vi "Open Base System Definition.vi"(8 "error in (no error)":errorcluster) -> (0 "error out":errorcluster, 2 "EST Custom Device":refnum<k24>, 3 "SystemDefinition":refnum<k24>)   [LabVIEW 2019, in "Engine Simulation Scripting API System Tests.lvclass"]
uses:
  Engine Simulation Scripting API System Tests.lvclass
  <vilib>/NI/VeriStand Custom Device Testing Tools/VeriStandTestUtilities/VeriStandTestUtilities.lvlib
  <userlib>/_OpenG.lib/file/file.llb/Append Path to Root if Relative - Scalar__ogtk.vi
  NationalInstruments.VeriStand.SystemDefinitionAPI
  Scripting API/Engine Simulation Toolkit Scripting API.lvlib
  Scripting API/Custom Device/Engine Simulation Toolkit Custom Device Settings.ctl
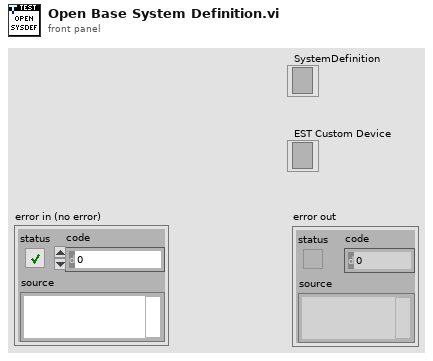
[diagram p1: front panel]
types:
  T1 = typedef "Engine Simulation Toolkit Scripting API.lvlib/Engine Simulation Toolkit Custom Device Settings.ctl" = cluster{"Name":string, "Execution priority":enum16{"Low", "Medium", "High"}, "Rate decimation":i32, "CPU":i32}
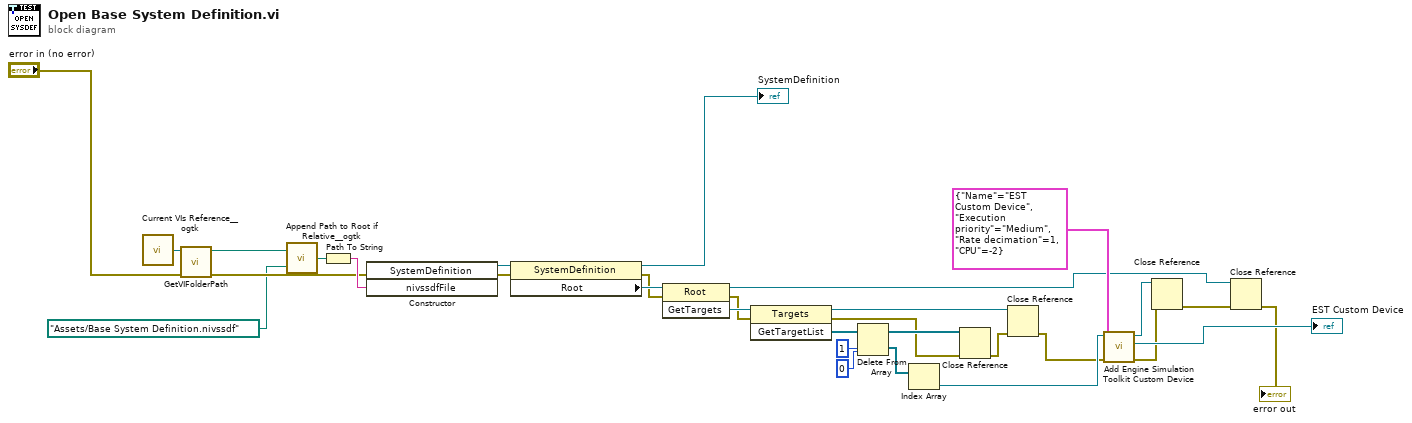
[diagram p0: block diagram]
diagram:
  n1 = call <userlib>:"Current VIs Reference__ogtk.vi"() -> ("Current VI's reference"=w8:refnum<vi>)  [unwired: 5 in]
  n2 = call <vilib>:"GetVIFolderPath.vi"("error in (no error)"="error in (no error)", "VI Reference in"=w8) -> ("error out"=w12:errorcluster, "VI Folder Path out"=w9:path)  [unwired: 8 in]
  n3 = call-poly <userlib>:"Append Path to Root if Relative__ogtk.vi"("Absolute or Relative Path"=path "Assets/Base System Definition.nivssdf", "Root Path"=w9) -> ("Absolute or Appended Path"=w11:path)
  n4 = Path To String(path=w11) -> (string=w14:string)
  n5 = constructor class="SystemDefinition"(error in=w12, "nivssdfFile"=w14) -> (reference out=w15:refnum<k24>, error out=w13:errorcluster)  [unwired: 2 in, 2 out]
  n6 = property class="SystemDefinition"(reference=w15, error in=w13) -> (reference out=→"SystemDefinition":refnum<k24>, error out=w16:errorcluster, "Root"=w17:refnum<k24>)
  n7 = invoke class="Root" method="GetTargets"(reference=w17, error in=w16) -> (reference out=w1:refnum<k24>, error out=w18:errorcluster, "GetTargets"=w19:refnum<k24>)  [unwired: 1 in]
  n8 = invoke class="Targets" method="GetTargetList"(reference=w19, error in=w18) -> (reference out=w26:refnum<k24>, error out=w23:errorcluster, "GetTargetList"=w20:refnum<k24>[])  [unwired: 1 in]
  n9 = Delete From Array(array=w20, length=1, index=0) -> (deleted portion=w27:refnum<k24>[], array with subset deleted=w24:refnum<k24>[])
  n10 = Index Array(array=w27) -> (element=w30:refnum<k24>)  [unwired: 1 in]
  n11 = Close Reference(reference=w24, error in (no error)=w23) -> (error out=w25:errorcluster)
  n12 = Close Reference(reference=w26, error in (no error)=w25) -> (error out=w29:errorcluster)
  n13 = call "Add Engine Simulation Toolkit Custom Device.vi"("error in (no error)"=w29, "Settings"=T1 {"Name"="EST Custom Device", "Execution priority"=enum."Medium", "Rate decimation"=1, "CPU"=-2}, "Target in"=w30) -> ("error out"=w6:errorcluster, "EST Custom Device"=→"EST Custom Device":refnum<k24>, "Target out"=w5:refnum<k24>)  [unwired: 6 in]
  n14 = Close Reference(reference=w5, error in (no error)=w6) -> (error out=w3:errorcluster)
  n15 = Close Reference(reference=w1, error in (no error)=w3) -> (error out=→"error out":errorcluster)
